vi "AIT 1553 - Clear Database - Dynamic.vi"(8 "error in (no error)":errorcluster, 11 "Node Ptr":u64 format="%.0x") -> (0 "error out":errorcluster)   [LabVIEW 2013]
uses:
  Controls and Global/Global.vi
  <vilib>/NI Veristand/Custom Device Tools/Custom Device Utility Library/NI VeriStand - Search for Item by GUID.vi
  <vilib>/NI Veristand/Custom Device API/Custom Device API.lvlib
  AIT 664 Custom Device.lvlib
  <vilib>/NI Veristand/Custom Device Tools/Custom Device Utility Library/Custom Device Utility Library.lvlib
panel:
  in  "Tag":string
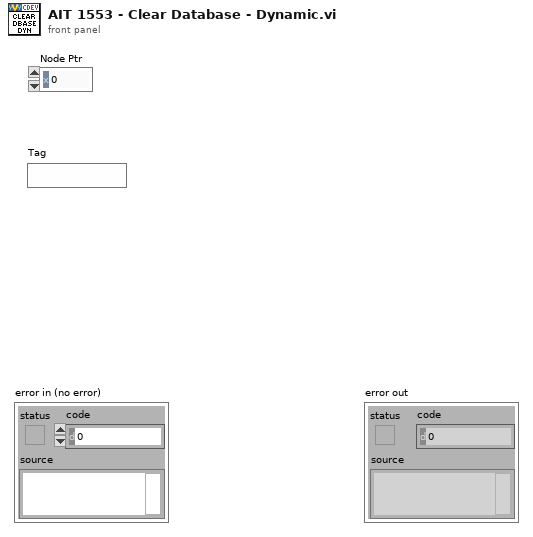
[diagram p1: front panel]
types:
  T1 = typedef "Custom Device API.lvlib/Custom Device Item Ref.ctl" = u64
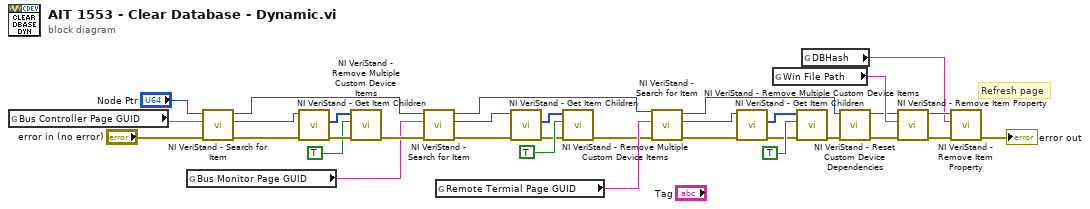
[diagram p0: block diagram]
diagram:
  # "Refresh page"
  n1 = global read "Global.vi" "Bus Controller Page GUID"() -> (w27:string)
  n2 = global read "Global.vi" "Bus Monitor Page GUID"() -> (w2:string)
  n3 = call-poly <vilib>:"NI VeriStand - Search for Item.vi"("error in"="error in (no error)", "Item GUID"=w27, "Section Ref in"="Node Ptr") -> ("error out"=w22:errorcluster, "Item Ref"=w25:T1, "Section Ref out"=w10:T1)  [unwired: 5 in, 1 out]
  n4 = call <vilib>:"NI VeriStand - Get Item Children.vi"("error in (no error)"=w22, "Item Ref in"=w25) -> ("error out"=w33:errorcluster, "Child Refs"=w28:T1[])  [unwired: 6 in, 2 out]
  n5 = call <vilib>:"NI VeriStand - Remove Multiple Custom Device Items.vi"("error in (no error)"=w33, "Force Delete (F)"=TRUE, "Item Refs in"=w28) -> ("error out"=w11:errorcluster)  [unwired: 7 in, 1 out]
  n6 = call-poly <vilib>:"NI VeriStand - Search for Item.vi"("error in"=w11, "Item GUID"=w2, "Section Ref in"=w10) -> ("error out"=w5:errorcluster, "Item Ref"=w3:T1, "Section Ref out"=w9:T1)  [unwired: 5 in, 1 out]
  n7 = global read "Global.vi" "Remote Termial Page GUID"() -> (w12:string)
  n8 = call <vilib>:"NI VeriStand - Get Item Children.vi"("error in (no error)"=w5, "Item Ref in"=w3) -> ("error out"=w6:errorcluster, "Child Refs"=w8:T1[])  [unwired: 6 in, 2 out]
  n9 = call <vilib>:"NI VeriStand - Remove Multiple Custom Device Items.vi"("error in (no error)"=w6, "Force Delete (F)"=TRUE, "Item Refs in"=w8) -> ("error out"=w4:errorcluster)  [unwired: 7 in, 1 out]
  n10 = call-poly <vilib>:"NI VeriStand - Search for Item.vi"("error in"=w4, "Item GUID"=w12, "Section Ref in"=w9) -> ("error out"=w20:errorcluster, "Item Ref"=w21:T1, "Section Ref out"=w14:T1)  [unwired: 5 in, 1 out]
  n11 = call <vilib>:"NI VeriStand - Get Item Children.vi"("error in (no error)"=w20, "Item Ref in"=w21) -> ("error out"=w23:errorcluster, "Child Refs"=w13:T1[])  [unwired: 6 in, 2 out]
  n12 = global read "Global.vi" "Win File Path"() -> (w30:string)
  n13 = call <vilib>:"NI VeriStand - Remove Multiple Custom Device Items.vi"("error in (no error)"=w23, "Force Delete (F)"=TRUE, "Item Refs in"=w13) -> ("error out"=w19:errorcluster)  [unwired: 7 in, 1 out]
  n14 = global read "Global.vi" "DBHash"() -> (w16:string)
  n15 = call <vilib>:"NI VeriStand - Reset Custom Device Dependencies.vi"("error in (no error)"=w19, "Device Ref in"=w14) -> ("error out"=w31:errorcluster, "Device Ref out"=w29:T1)  [unwired: 8 in]
  n16 = call <vilib>:"NI VeriStand - Remove Item Property.vi"("error in (no error)"=w31, "Property Name"=w30, "Item Ref in"=w29) -> ("error out"=w18:errorcluster, "Item Ref out"=w17:T1)  [unwired: 6 in, 1 out]
  n17 = call <vilib>:"NI VeriStand - Remove Item Property.vi"("error in (no error)"=w18, "Property Name"=w16, "Item Ref in"=w17) -> ("error out"=→"error out":errorcluster)  [unwired: 6 in, 2 out]
